vi "02 ListenLoop.vi"(8 "error in (no error)":errorcluster caption="错误输入（无错误）", 10 "超时毫秒":i32, 11 "TCPServerClass 输入":refnum<class "TCPServerClass.lvclass">) -> (0 "error out":errorcluster caption="错误输出", 2 "新增":bool, 3 "TCPServerClass 输出":refnum<class "TCPServerClass.lvclass">)   [LabVIEW 2019, in "TCPServerClass.lvclass"]
uses:
  TCPServerClass.lvclass
  TCPServerClass.lvclass/TCPServerClass.ctl
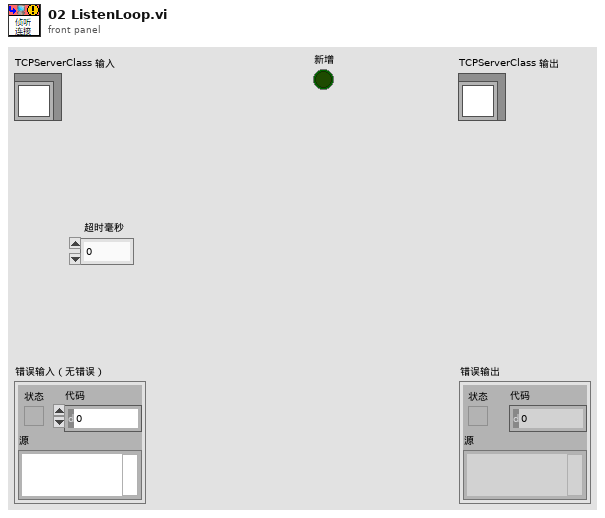
[diagram p1: front panel]
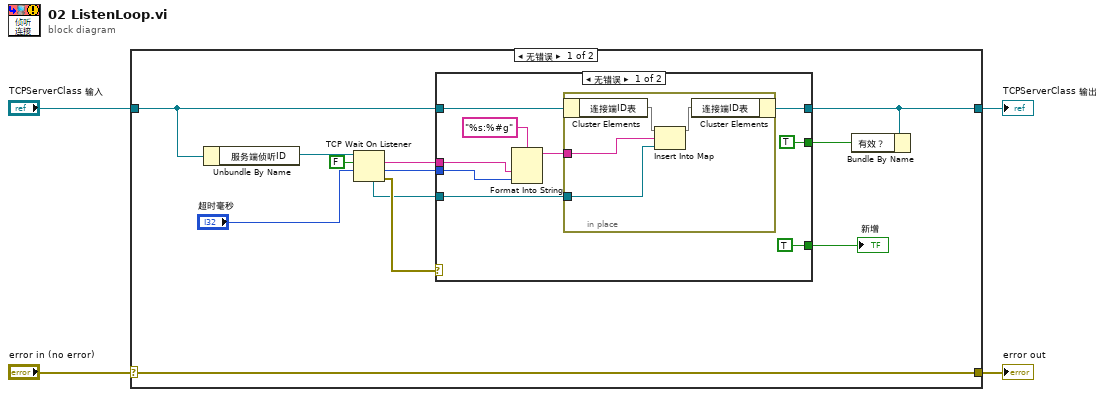
[diagram p0: block diagram]
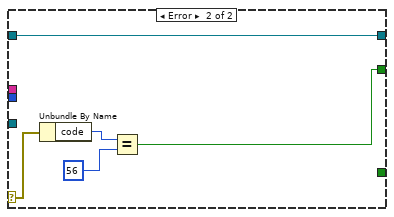
[diagram p2: hidden frame]
diagram:
  n1 = case shown="无错误" "error in (no error)" {
    selector: "error in (no error)" -> [w16 w36]
    tunnel: [w16 w36] -> w3
    tunnel: [w10 w35] -> w1
    tunnel: "TCPServerClass 输入" -> [w11 w35]
    frame No Error {
      n2 = Unbundle By Name(w11) -> ("服务端侦听ID"=w15:refnum<k5>)
      n3 = TCP Wait On Listener(9:"超时毫秒", 10:FALSE ("解析远程地址(T)"), 11:w15) -> (0:w12:errorcluster, 1:w6:u16, 2:w7:string, 4:w8:refnum<k5>)  [unwired: 1 in, 1 out]
      n4 = case shown="无错误" w12 {
        selector: w12 -> [_ w33]
        tunnel: [w23 w34] -> w10
        tunnel: w11 -> [w24 w34]
        tunnel: [TRUE w30] -> w9
        tunnel: w8 -> [w22 _]
        tunnel: w7 -> [w20 _]
        tunnel: w6 -> [w19 _]
        tunnel: [TRUE _] -> w5
        frame No Error {
          n5 = Format Into String(format string="%s:%#g" ("格式字符串"), w20, w19) -> (resulting string=w18:string)  [unwired: 2 in, 1 out]
          n6 = in-place {
            in-place-border: w22 -> [w27]
            in-place-border: w18 -> [w26]
            n7 = in-place-cluster #1(w24) -> ("连接端ID表"=w29:map{string, refnum<k5>})
            n8 = Insert Into Map(map in=w29, key=w26, value=w27) -> (map out=w28:map{string, refnum<k5>})  [unwired: 2 out]
            n9 = in-place-cluster #1("连接端ID表"=w28) -> (w23:refnum<class "TCPServerClass.lvclass">)
          }
        }
        frame Error {
          n10 = Unbundle By Name(w33) -> ("code"=w32:i32)
          n11 = Equal?(x=w32, y=56) -> (x = y?=w30:bool)
        }
      }
      "新增" <- w5
      n12 = Bundle By Name(cluster=w10, "有效？"=w9) -> ()  [unwired: 1 out]
    }
    frame Error {
    }
  }
  "error out" <- w3
  "TCPServerClass 输出" <- w1
